vi "All Node Groups.vi"(8 "error in (no error)":errorcluster, 10 "Node Name":string, 11 "ChannelService in":refnum<class "ChannelService.lvclass">) -> (0 "error out":errorcluster, 2 "Node Groups":refnum<class "GroupAbstract.lvclass">[](array[class]), 3 "ChannelService out":refnum<class "ChannelService.lvclass">)   [LabVIEW 2020, in "Vecto.lvlib" / "ChannelService.lvclass"]
uses:
  ChannelService.lvclass
  ChannelService.lvclass/ChannelService.ctl
  GroupsAbstractValue/GroupsAbstractValue.lvclass
  lv-promises/Promises/Future/Future.lvclass
  lv-promises/Promises/Promise/Promise.lvclass
  C:/dev/lv20CE/relink/lv-promises/Promises/Value/Value.lvclass
  C:/dev/lv20CE/relink/lv-vecto/Vecto/GroupsAbstractValue/GroupsAbstractValue.lvclass
  Node Groups Data.ctl
  GroupAbstract/GroupAbstract.lvclass
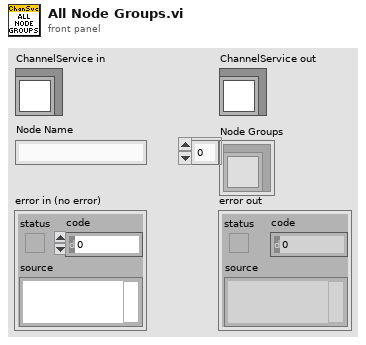
[diagram p1: front panel]
types:
  T1 = typedef "Vecto.lvlib/ChannelService.lvclass/Node Groups Data.ctl" = cluster{"Node Name":string, "Promise":refnum<class "Promise.lvclass">}
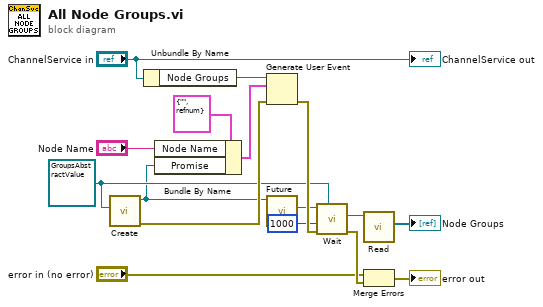
[diagram p0: block diagram]
diagram:
  w10 = refnum<class "GroupsAbstractValue.lvclass"> refnum ("Vecto.lvlib:GroupsValue.lvclass")
  n1 = call "Create.vi"("Result Type"=w10) -> ("error out"=w13:errorcluster, "Promise"=w5:refnum<class "Promise.lvclass">)  [unwired: 9 in]
  n2 = Unbundle By Name("ChannelService in") -> ("Node Groups"=w12:refnum<user-event>)
  n3 = Bundle By Name(cluster=T1 {"Node Name"="", "Promise"=refnum} ("Node Groups Data"), "Node Name"="Node Name", "Promise"=w5) -> (w4:T1)
  n4 = Generate User Event(user event=w12, event data cluster=w4, error in=w13) -> (error out=w14:errorcluster)  [unwired: 1 in, 1 out]
  n5 = call "Future.vi"("Promise in"=w5) -> ("Future"=w11:refnum<class "Future.lvclass">)  [unwired: 9 in, 1 out]
  n6 = call "Wait.vi"("Result Type"=w10, "error in (no error)"=w14, "Timeout mS (-1)"=1000, "Future in"=w11) -> ("error out"=w16:errorcluster, "Result"=w8:refnum<class "GroupsAbstractValue.lvclass">)  [unwired: 6 in]
  n7 = call "Read.vi"("GroupsAbstractValue in"=w8) -> ("Groups"=→"Node Groups":refnum<class "GroupAbstract.lvclass">[])  [unwired: 10 in]
  n8 = Merge Errors("error in (no error)", w16) -> (→"error out":errorcluster)
  "ChannelService out" <- "ChannelService in"
